vi "Color Chooser Update.vi"(5 "Color Chooser":enum16{"unchanged", "Color Box", "Color List"}(ring)) -> (0 "Color Box Visible":bool, 1 "Color List Visible":bool)   [LabVIEW 2019]
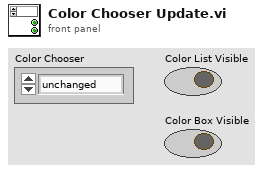
[diagram p1: front panel]
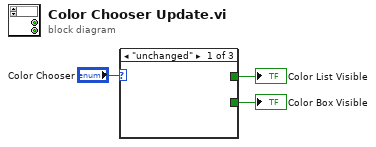
[diagram p0: block diagram]
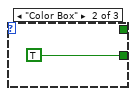
[diagram p2: hidden frame]
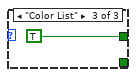
[diagram p3: hidden frame]
diagram:
  n1 = case shown="\"unchanged\"" "Color Chooser" {
    tunnel: [_ _ TRUE ("Visible")] -> w2
    tunnel: [_ TRUE ("Visible") _] -> w3
    frame "unchanged" {
    }
    frame "Color Box" {
    }
    frame "Color List" {
    }
  }
  "Color Box Visible" <- w3
  "Color List Visible" <- w2
